vi "Do This.vi"(8 "error in (no error)":errorcluster, 10 "Status Events":refnum<class "Status Events.lvclass">, 11 "Dummy Job in":refnum<class "Dummy Job.lvclass">) -> (0 "error out":errorcluster, 3 "Dummy Job out":refnum<class "Dummy Job.lvclass">)   [LabVIEW 2014, in "Dummy Job.lvclass"]
uses:
  Dummy Job.lvclass
  Core/Shared/Classes/Status Events/Status Events.lvclass
  Dummy Job.lvclass/Dummy Job.ctl
  Core/LabVIEW CI Service/Classes/Job/Job.lvclass/Job.ctl
  Core/LabVIEW CI Service/Classes/Job/Job.lvclass
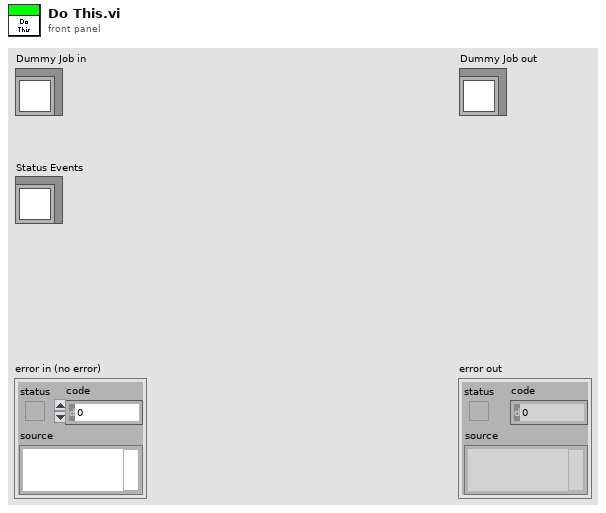
[diagram p1: front panel]
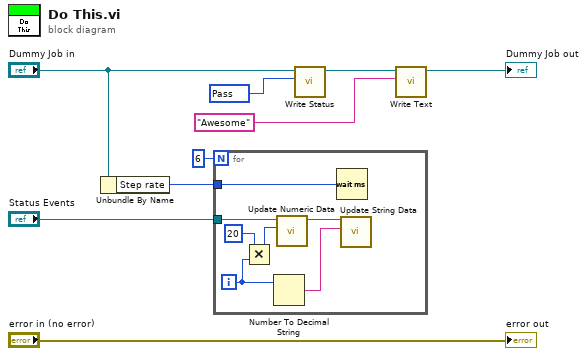
[diagram p0: block diagram]
diagram:
  w6 = u16 200 items=["Service Error"=504, "Abort"=503, "Fail"=500, "Pass"=200] ("Status")
  n1 = Unbundle By Name("Dummy Job in") -> ("Step rate"=w2:u32)
  n2 = for {
    N: 6 -> [_]
    tunnel: "Status Events" -> [w15]
    tunnel: w2 -> [w14]
    i -> [w11]
    n3 = Multiply(x=20, y=w11) -> (x*y=w12:i32)
    n4 = Number To Decimal String(number=w11) -> (decimal integer string=w10:string)  [unwired: 1 in]
    n5 = call "Update Numeric Data.vi"("Numeric Data"=w12, "Status Updater in"=w15) -> ("Status Updater out"=w16:refnum<class "Status Events.lvclass">)  [unwired: 8 in, 1 out]
    n6 = Wait (ms)(milliseconds to wait=w14) -> ()  [unwired: 1 out]
    n7 = call "Update String Data.vi"("String Data"=w10, "Status Updater in"=w16) -> ()  [unwired: 8 in, 2 out]
  }
  n8 = call "Write Status.vi"("Status"=w6, "Job in"="Dummy Job in") -> ("Job out"=w8:refnum<class "Dummy Job.lvclass">)  [unwired: 8 in, 1 out]
  n9 = call "Write Text.vi"("Text"="Awesome", "Job in"=w8) -> ("Job out"=→"Dummy Job out":refnum<class "Dummy Job.lvclass">)  [unwired: 8 in, 1 out]
  "error out" <- "error in (no error)"
